vi "Measurement Array Process.vi"(11 "Image Cluster Input":T2={"Results and Tolerance \nLimits 2D array"=[], "Measurement Names Array"=[], "Image Array"=["Result", "Tolerance Limits"], "Measurement Values Array"=[], "Images_Array_in"=[], "Tolerance  Array"=[]}) -> (3 "Array out":string[][](array[string]))   [LabVIEW 2015, in "ZenGage v3.0 UI.lvclass"]
uses:
  ZenGage v3.0 UI.lvclass
  <vilib>/vision/Image Controls.llb/IMAQ Image.ctl
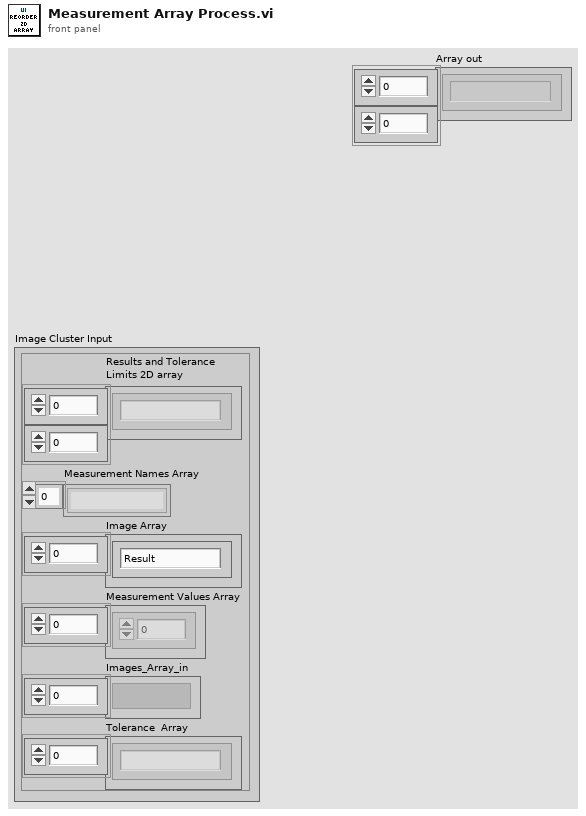
[diagram p1: front panel]
types:
  T1 = typedef "IMAQ Image.ctl" = refnum<image>
  T2 = cluster{"Results and Tolerance \nLimits 2D array":string[][], "Measurement Names Array":string[], "Image Array":string[], "Measurement Values Array":dbl[], "Images_Array_in":T1[], "Tolerance  Array":string[]}
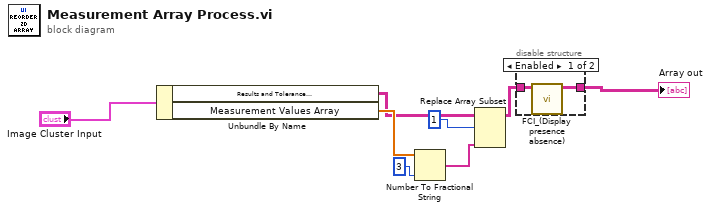
[diagram p0: block diagram]
diagram:
  n1 = Unbundle By Name("Image Cluster Input") -> ("Results and Tolerance \nLimits 2D array"=w6:string[][], "Measurement Values Array"=w7:dbl[])
  n2 = Number To Fractional String(number=w7, precision (6)=i16 3) -> (F-format string=w1:string[])  [unwired: 2 in]
  n3 = Replace Array Subset(array=w6, new element=w1, index (row)=1) -> (w5:string[][])  [unwired: 1 in]
  n4 = disable-structure shown="Enabled" {
    disable-tunnel: w5 -> [w10 w11]
    disable-tunnel: [w9 w11] -> w3
    frame Enabled {
      n5 = call "FCI_(Display presence absence).vi"("Display Array"=w10) -> ("Display Array"=w9:string[][])  [unwired: 10 in]
    }
    frame Disabled {
    }
  }
  "Array out" <- w3
